vi "define.vi"(8 "error in (no error)":errorcluster, 11 "TrajectoryTS090820Circular2D in":refnum<class "TrajectoryTS090820Circular2D.lvclass">) -> (0 "error out":errorcluster, 3 "TrajectoryTS090820Circular2D out":refnum<class "TrajectoryTS090820Circular2D.lvclass">)   [LabVIEW 2010, in "TrajectoryTS090820Circular2D.lvclass"]
uses:
  TrajectoryTS090820Circular2D.lvclass
  trajectory_type_enum.ctl
  TrajectoryTS090820Circular2D.lvclass/TrajectoryTS090820Circular2D.ctl
  common/classes/Image/Image/Image.lvclass
panel:
  in  "trajectory type":T1
  in  "cancelButton":bool
  in  "acceptButton":bool
  in  "load image button":bool
  in  "y center":dbl
  in  "x center":dbl
  in  "rotation angle":dbl
  in  "spiral?":bool
  in  "dump factor":dbl=1.1
  in  "y amplitude":dbl[unit]=9.999999999999999e-06
  in  "x frequency":dbl=1.0
  in  "y frequency":dbl=1.0
  in  "phase shift":dbl
  in  "number of pixels per cycle":i32=250 min=0
  in  "x amplitude":dbl[unit]=9.999999999999999e-06
  in  "Double":bool
  out "reference image":T2(plugin-control)
  # "Define trajectory"
  # "trajectory parameters"
  # "spiral"
  # "centering"
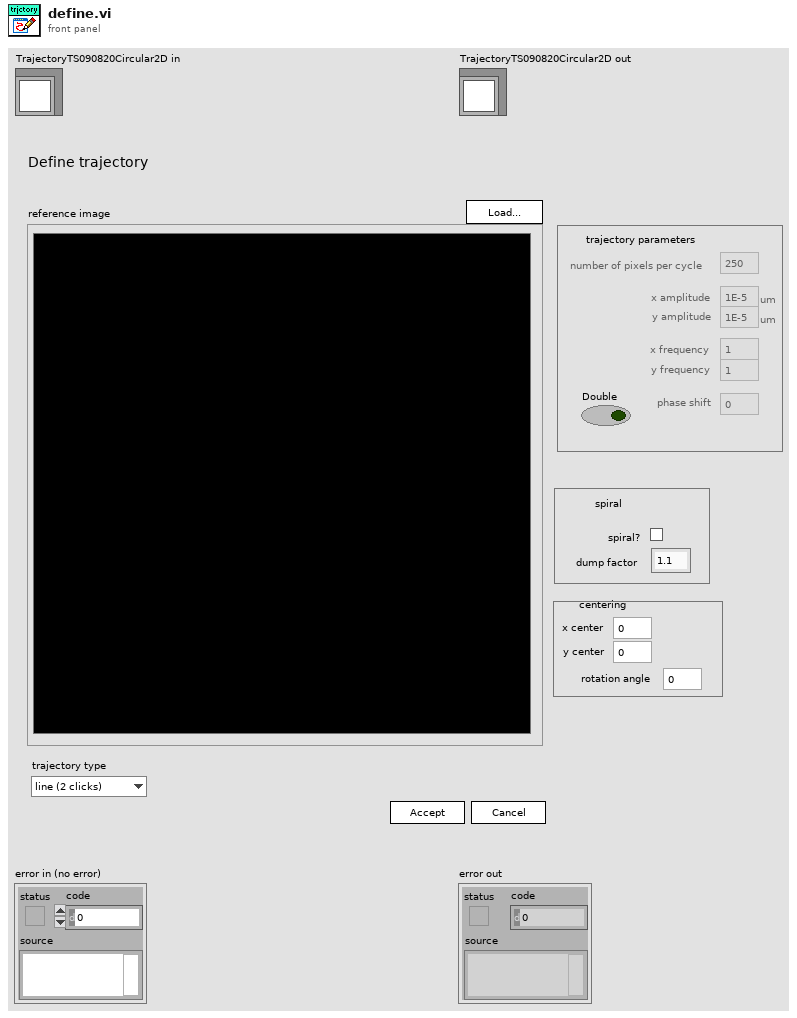
[diagram p1: front panel]
types:
  T1 = typedef "trajectory_type_enum.ctl" = enum16{"line (2 clicks)", "circular (2 clicks)", "elliptical (3 clicks)", "double circle (3 clicks)"}
  T2 = typedef "IMAQ Image.ctl" = refnum<image>
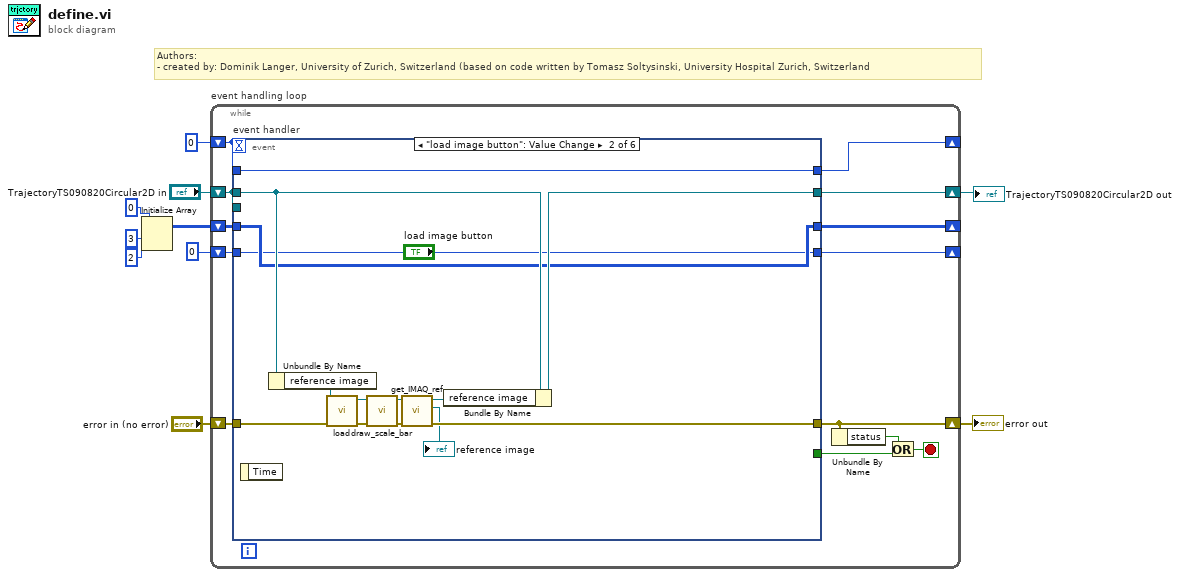
[diagram p0: block diagram]
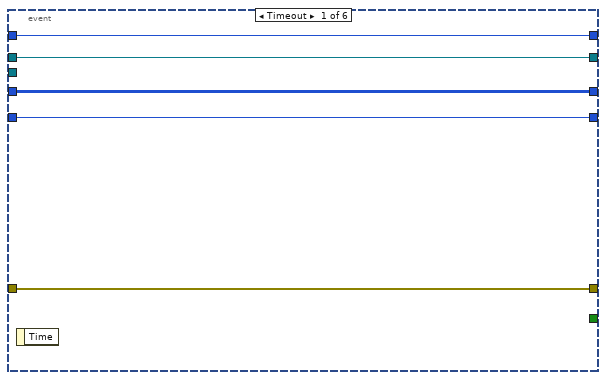
[diagram p2: hidden frame]
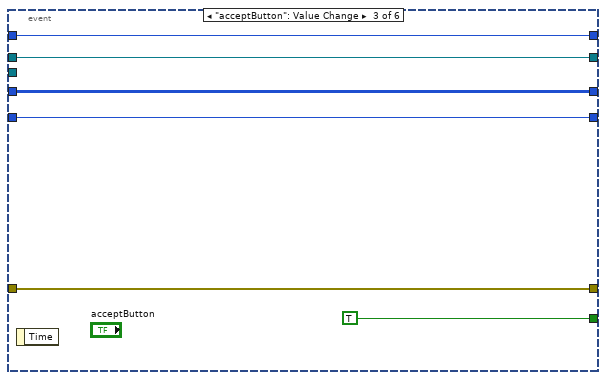
[diagram p3: hidden frame]
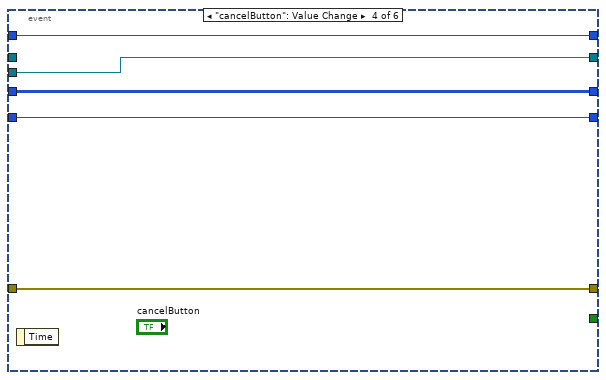
[diagram p4: hidden frame]
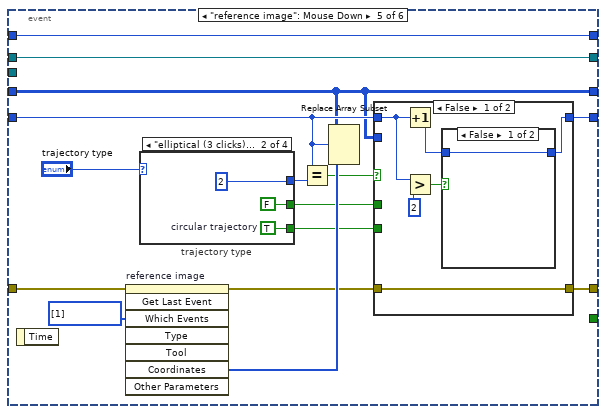
[diagram p5: hidden frame]
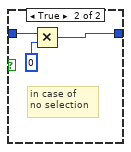
[diagram p6: hidden frame]
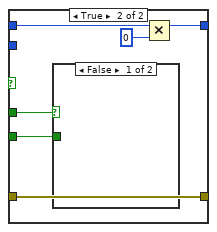
[diagram p7: hidden frame]
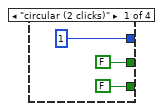
[diagram p9: hidden frame]
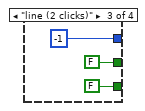
[diagram p10: hidden frame]
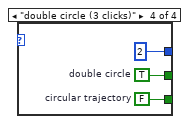
[diagram p11: hidden frame]
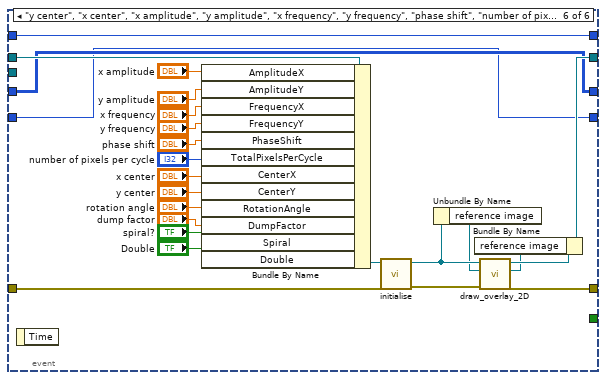
[diagram p12: hidden frame]
diagram:
  # "Authors: \n- created by: Dominik Langer, University of Zurich, Switzerland (based on code written by Tomasz Soltysinski, University Hospital Zurich, Switzerland"
  n1 = Initialize Array(0, 3 ("dimension size"), 2 ("dimension size")) -> (w1:i32[][])
  n2 = while "event handling loop" {
    shift-right: [w22] -> _
    shift-left: 0 -> [w23]
    shift-right: [w19] -> w8
    shift-left: "error in (no error)" -> [w21]
    shift-right: [w20] -> w6
    shift-left: "TrajectoryTS090820Circular2D in" -> [w15]
    shift-right: [w13] -> _
    shift-left: w1 -> [w14]
    shift-right: [w12] -> _
    shift-left: 0 -> [w11]
    stop <- w16 stop-if-true
    n3 = event "event handler" shown="[1] \"load image button\": Value Change" {
      selector: _ -> [_ _ _ _ _ _]
      dyn-events: _ -> [_ _ _ _ _ _]
      timeout: w23 -> [_ _ _ _ _ _]
      tunnel: [w28 w42 w48 w53 w68 w121] -> w22
      tunnel: w23 -> [w28 w42 w48 w53 w68 w121]
      tunnel: w21 -> [w27 w36 w47 w52 w65 w116]
      tunnel: [w27 w35 w47 w52 w56 w115] -> w19
      tunnel: w15 -> [w26 w33 w46 _ w67 w120]
      tunnel: [w26 w32 w46 w51 w67 w109] -> w20
      tunnel: [_ _ TRUE _ _ _] -> w17
      tunnel: w15 -> [_ _ _ w51 _ _]
      tunnel: w14 -> [w25 w30 w44 w50 w55 w108]
      tunnel: [w25 w30 w44 w50 w55 w108] -> w13
      tunnel: w11 -> [w24 w29 w43 w49 w59 w107]
      tunnel: [w24 w29 w43 w49 w58 w107] -> w12
      event Timeout {
        n4 = event-data() -> ()  [unwired: 1 in, 1 out]
      }
      event "load image button": Value Change {
        n5 = event-data() -> ()  [unwired: 1 in, 1 out]
        n6 = Unbundle By Name(w33) -> ("reference image"=w41:refnum<class "Image.lvclass">)
        n7 = call-dynamic "load.vi"("error in (no error)"=w36, "Image in"=w41) -> ("error out"=w40:errorcluster, "Image out"=w38:refnum<class "Image.lvclass">)  [unwired: 6 in, 2 out]
        n8 = call "draw_scale_bar.vi"("error in (no error)"=w40, "Image in"=w38) -> ("error out"=w39:errorcluster, "Image out"=w37:refnum<class "Image.lvclass">)  [unwired: 8 in]
        n9 = call-dynamic "get_IMAQ_ref.vi"("error in (no error)"=w39, "Image.lvclass in"=w37) -> ("error out"=w35:errorcluster, "Image"=→"reference image":T2, "Image.lvclass out"=w34:refnum<class "Image.lvclass">)  [unwired: 5 in, 2 out]
        n10 = Bundle By Name(cluster=w33, "reference image"=w34) -> (w32:refnum<class "TrajectoryTS090820Circular2D.lvclass">)
      }
      event "acceptButton": Value Change {
        n11 = event-data() -> ()  [unwired: 1 in, 1 out]
      }
      event "cancelButton": Value Change {
        n12 = event-data() -> ()  [unwired: 1 in, 1 out]
      }
      event "reference image": Mouse Down {
        w66 = i32[] [1] items=["No  event", "Click event", "Draw event", "Move event", "Size event", "Scroll event", "Activate event", "Close event", "Double click event"] ("Events list (all)")
        n13 = event-data() -> ()  [unwired: 1 in, 1 out]
        n14 = invoke on="reference image" class="ImageControl" method="Get Last Event"(error in=w65, "Which Events"=w66) -> (error out=w57:errorcluster, "Coordinates"=w64:i32[])  [unwired: 6 in, 6 out]
        n15 = case "trajectory type" shown="\"elliptical (3 clicks)\"" "trajectory type" {
          tunnel: [1 2 -1 2] -> w63
          tunnel: [FALSE w89 FALSE ("circular trajectory") w95] -> w60
          tunnel: [FALSE ("double circle") FALSE ("double circle") FALSE ("double circle") w94] -> w61
          frame "circular (2 clicks)" {
          }
          frame "elliptical (3 clicks)" {
            w89 = TRUE  # circular trajectory
          }
          frame "line (2 clicks)" {
          }
          frame "double circle (3 clicks)" {
            w94 = TRUE  # double circle
            w95 = FALSE  # circular trajectory
          }
        }
        n16 = Equal?(x=w59, y=w63) -> (x = y?=w62:bool)
        n17 = Replace Array Subset(array=w55, new element=w64, index (row)=w59) -> ()  [unwired: 1 in, 1 out]
        n18 = case shown="False" w62 {
          tunnel: w61 -> [_ w80]
          tunnel: w60 -> [_ w79]
          tunnel: w59 -> [w72 w82]
          tunnel: [w69 w81] -> w58
          tunnel: w57 -> [w74 w84]
          tunnel: [w74 w84] -> w56
          tunnel: w55 -> [_ _]
          frame False {
            n19 = Increment(x=w72) -> (x+1=w70:i32)
            n20 = Greater?(x=w72, y=2) -> (0:w71:bool)
            n21 = case shown="False" w71 {
              tunnel: w70 -> [w75 w77]
              tunnel: [w75 w76] -> w69
              frame False {
              }
              frame True {
                # "in case of\nno selection"
                n22 = Multiply(x=w77, y=0 ("x")) -> (x*y=w76:i32)
              }
            }
          }
          frame True {
            n23 = case shown="False" w80 {
              tunnel: w79 -> [_ _]
              frame False {
              }
              frame True {
              }
            }
            n24 = Multiply(x=w82, y=0) -> (x*y=w81:i32)
          }
        }
      }
      event "y center", "x center", "x amplitude", "y amplitude", "x frequency", "y frequency", "phase shift", "number of pixels per cycle", "rotation angle", "spiral?", "dump factor", "Double": Value Change {
        n25 = event-data() -> ()  [unwired: 1 in, 1 out]
        n26 = Bundle By Name(cluster=w120, "AmplitudeX"="x amplitude", "AmplitudeY"="y amplitude", "FrequencyX"="x frequency", "FrequencyY"="y frequency", "PhaseShift"="phase shift", "TotalPixelsPerCycle"="number of pixels per cycle", "CenterX"="x center", "CenterY"="y center", "RotationAngle"="rotation angle", "DumpFactor"="dump factor", "Spiral"="spiral?", "Double"="Double") -> (w110:refnum<class "TrajectoryTS090820Circular2D.lvclass">)
        n27 = call-dynamic "initialise.vi"("error in (no error)"=w116, "TrajectoryTS090820Circular2D in"=w110) -> ("error out"=w117:errorcluster, "TrajectoryTS090820Circular2D out"=w114:refnum<class "TrajectoryTS090820Circular2D.lvclass">)  [unwired: 8 in]
        n28 = Unbundle By Name(w114) -> ("reference image"=w113:refnum<class "Image.lvclass">)
        n29 = call-dynamic "draw_overlay_2D.vi"("error in (no error)"=w117, "image in"=w113, "GenericTrajectory in"=w114) -> ("error out"=w115:errorcluster, "image out"=w111:refnum<class "Image.lvclass">, "GenericTrajectory out"=w112:refnum<class "TrajectoryTS090820Circular2D.lvclass">)  [unwired: 6 in]
        n30 = Bundle By Name(cluster=w112, "reference image"=w111) -> (w109:refnum<class "TrajectoryTS090820Circular2D.lvclass">)
      }
    }
    n31 = Unbundle By Name(w19) -> ("status"=w18:bool)
    n32 = Or(x=w18, y=w17) -> (x .or. y?=w16:bool)
  }
  "error out" <- w8
  "TrajectoryTS090820Circular2D out" <- w6
